vi "BRig_arrTrig_Cue2LED.vi"() -> (2 "output_Cue2LED":i32)   [LabVIEW 2014]
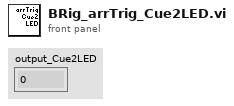
[diagram p1: front panel]
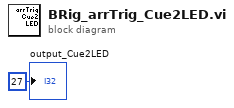
[diagram p0: block diagram]
diagram:
  "output_Cue2LED" <- 27
